vi "Wait.vi"(8 "error in (no error)":errorcluster, 10 "wait? (true)":bool=TRUE, 11 "milliseconds to wait":u32=200) -> (0 "error out":errorcluster)   [LabVIEW 2018]
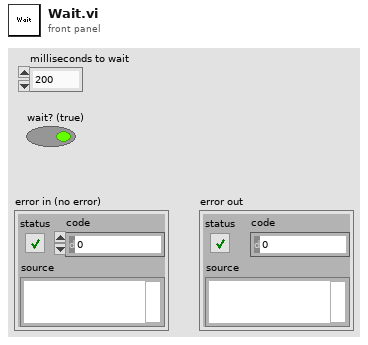
[diagram p1: front panel]
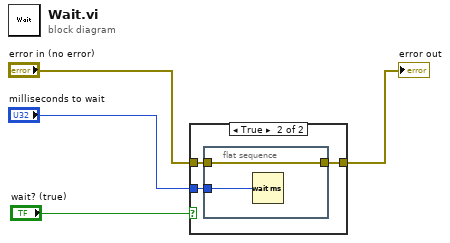
[diagram p0: block diagram]
diagram:
  n1 = case shown="True" "wait? (true)" {
    tunnel: [w5 w8] -> w4
    tunnel: "error in (no error)" -> [w5 w7]
    tunnel: "milliseconds to wait" -> [_ w6]
    frame False {
    }
    frame True {
      n2 = flat-sequence {
        tunnel: w7 -> [w10]
        tunnel: [w10] -> w8
        tunnel: w6 -> [w9]
        frame #0 {
          n3 = Wait (ms)(milliseconds to wait=w9) -> ()  [unwired: 1 out]
        }
      }
    }
  }
  "error out" <- w4
